vi "motorMoveVector.vi"(4 "Distance":sgl, 5 "Device in":refnum<k24>) -> (2 "Device out":refnum<k24>)   [LabVIEW 2014]
doc: "André Romero - 2017\nandretec@ifsc.usp.br"
uses:
  C:/users-lab/Andre/GITs/andretec/Thorlabs-Vector-Move/kinesisTec/Kinesis/Thorlabs.MotionControl.TCube.DCServoCLI.dll
  Kinesis/Thorlabs.MotionControl.TCube.DCServoCLI.dll
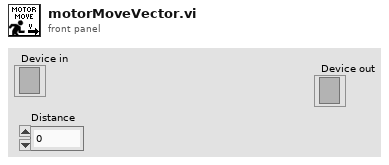
[diagram p1: front panel]
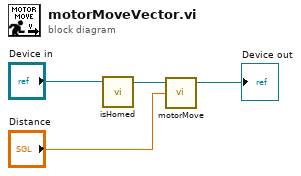
[diagram p0: block diagram]
diagram:
  n1 = call "isHomed.vi"("Device in"="Device in") -> ("Device out"=w3:refnum<k24>)  [unwired: 4 in]
  n2 = call "motorMove.vi"("position"="Distance", "Device in"=w3) -> ("Device out"=→"Device out":refnum<k24>)  [unwired: 3 in]
